vi "Humidity Write Single.vi"(8 "error in":errorcluster, 9 "Channel Index":i32=1, 10 "Humidity AV":dbl, 11 "Climate Chamber in":refnum<class "Climate Chamber.lvclass">) -> (0 "error out":errorcluster, 3 "Climate Chamber out":refnum<class "Climate Chamber.lvclass">)   [LabVIEW 2023, in "Climate Chamber.lvclass"]
uses:
  Climate Chamber.lvclass
  Climate Chamber.lvclass/Climate Chamber.ctl
  Low Level Capabilities/Humidity/Humidity Actual Value/Humidity Actual Value.lvclass
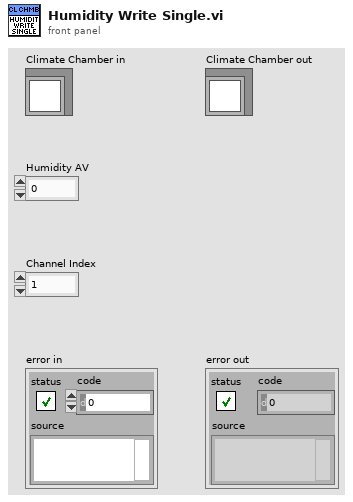
[diagram p1: front panel]
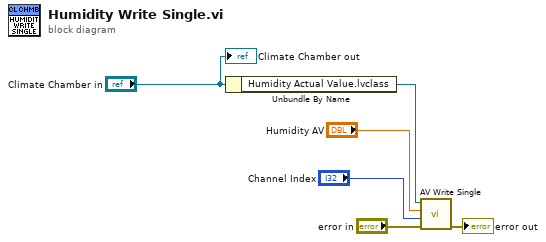
[diagram p0: block diagram]
diagram:
  n1 = Unbundle By Name("Climate Chamber in") -> ("Humidity Actual Value.lvclass"=w5:refnum<class "Humidity Actual Value.lvclass">)
  n2 = call-dynamic "AV Write Single.vi"("error in"="error in", "Channel Index"="Channel Index", "Humidity AV"="Humidity AV", "Humidity Actual Value in"=w5) -> ("error out"=→"error out":errorcluster)  [unwired: 6 in, 1 out]
  "Climate Chamber out" <- "Climate Chamber in"
